vi "Estimate Absolute Orientation.vi"   [LabVIEW 2020, in "pointset_utils.lvlib"]
uses:
  pointset_utils.lvlib
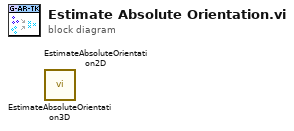
[diagram p0: block diagram]
diagram:
  n1 = call "EstimateAbsoluteOrientation3D.vi"() -> ()  [unwired: 7 in, 5 out]
  n2 = call "EstimateAbsoluteOrientation2D.vi"() -> ()  [unwired: 7 in, 5 out]
